vi "LogError.vi"(8 "error in (no error)":errorcluster, 11 "TCP_Server_Connection_Handler in":refnum<class "TCP_Server_Connection_Handler.lvclass">) -> (0 "error out":errorcluster, 3 "TCP_Server_Connection_Handler out":refnum<class "TCP_Server_Connection_Handler.lvclass">)   [LabVIEW 2023, in "TCP_Server_Connection_Handler.lvlib" / "TCP_Server_Connection_Handler.lvclass"]
uses:
  TCP_Server_Connection_Handler.lvclass
  TCP_Server_Connection_Handler.lvclass/TCP_Server_Connection_Handler.ctl
  SimpleErrorLogger/SimpleErrorLogger Messages/LogError Msg/LogError Msg.lvclass
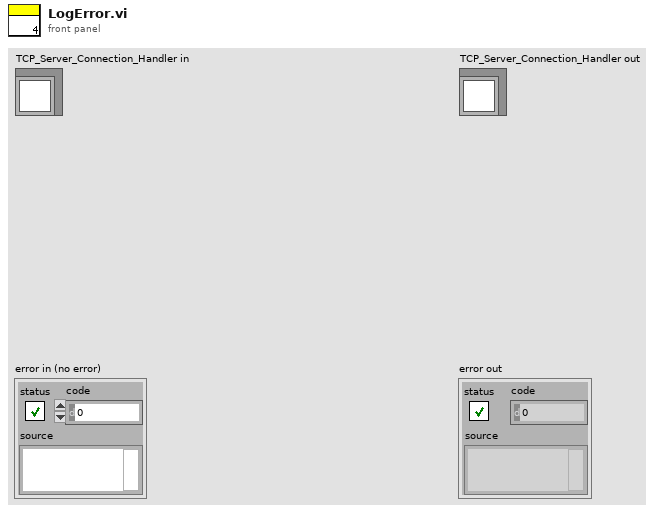
[diagram p1: front panel]
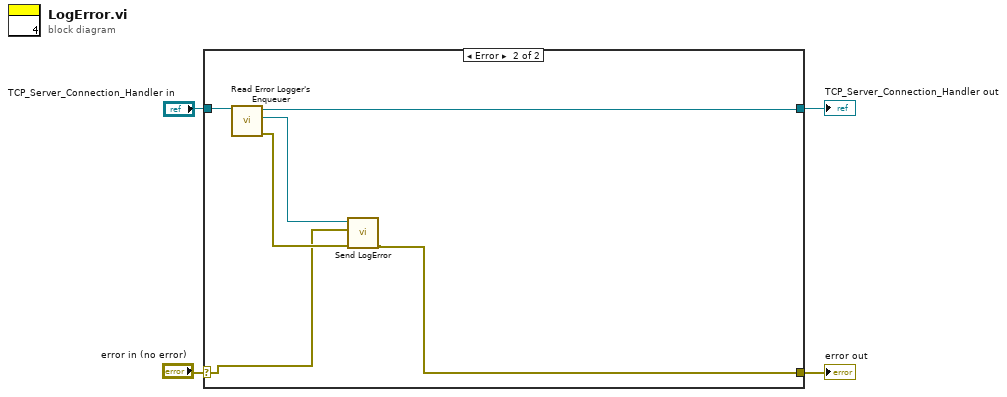
[diagram p0: block diagram]
diagram:
  n1 = case shown="Error" "error in (no error)" {
    selector: "error in (no error)" -> [w5 w9]
    tunnel: [w5 w7] -> w3
    tunnel: [w6 w11] -> w1
    tunnel: "TCP_Server_Connection_Handler in" -> [w6 w12]
    frame No Error {
    }
    frame Error {
      n2 = call "Read Error Logger's Enqueuer.vi"("TCP_Server_Connection_Handler in"=w12) -> ("error out"=w10:errorcluster, "Actor Framework:Message Enqueuer"=w8:refnum<class "Message Enqueuer.lvclass">, "TCP_Server_Connection_Handler out"=w11:refnum<class "TCP_Server_Connection_Handler.lvclass">)  [unwired: 8 in]
      n3 = call "Send LogError.vi"("error in (no error)"=w10, "error"=w9, "Message Enqueuer"=w8) -> ("error out"=w7:errorcluster)  [unwired: 7 in, 1 out]
    }
  }
  "error out" <- w3
  "TCP_Server_Connection_Handler out" <- w1
